vi "populate db with default.vi"(0 "SQLite Connection in":refnum<class "Connection.lvclass">, 7 "input pk list":string[](array[string]), 9 "table name":string, 11 "error in":errorcluster) -> (4 "SQLite Connection out":refnum<class "Connection.lvclass">, 15 "error out":errorcluster)   [LabVIEW 2014, in "SQLite runtime.lvclass"]
uses:
  SQLite runtime.lvclass
  <vilib>/drjdpowell/SQLite Library/SQL Connection/Connection.lvclass
  <vilib>/NI/Tag Bus/table/data table.ctl
  <vilib>/drjdpowell/SQLite Library/SQL Statement/SQL Statement.lvclass/SQL Statement.ctl
  <vilib>/drjdpowell/SQLite Library/SQL Statement/Bind Integer.vi
  <vilib>/drjdpowell/SQLite Library/SQL Statement/Bind Real.vi
  <vilib>/drjdpowell/SQLite Library/SQL Statement/Bind Text.vi
  <vilib>/drjdpowell/SQLite Library/SQL Statement/Step.vi
  <vilib>/drjdpowell/SQLite Library/SQL Statement/Error Message.vi
  <vilib>/drjdpowell/SQLite Library/SQL Statement/SQL Statement.lvclass
  <vilib>/NI/Tag Bus/table/data table.lvlib
panel:
  in  "data table":T1
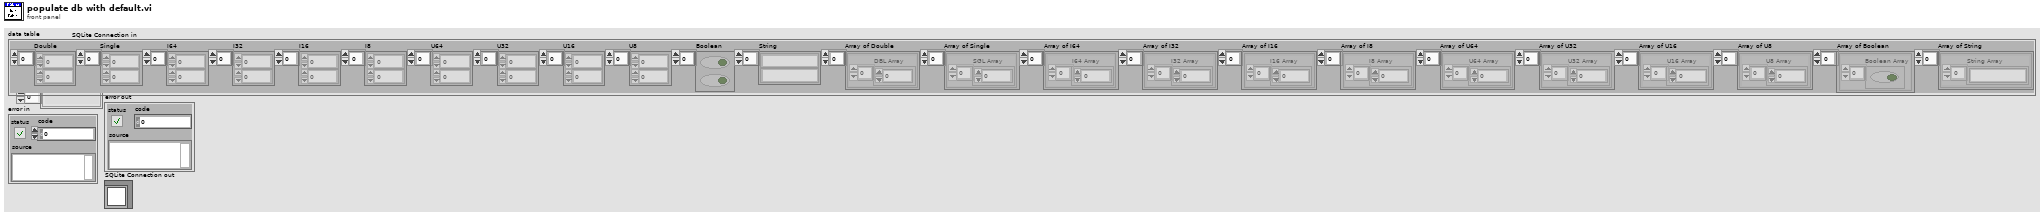
[diagram p1: front panel]
types:
  T1 = typedef "tag bus.lvlib/data table.lvlib/data table.ctl" = cluster{"Double":dbl[], "Single":sgl[], "I64":i64[], "I32":i32[], "I16":i16[], "I8":i8[], "U64":u64[], "U32":u32[], "U16":u16[], "U8":u8[], "Boolean":bool[], "String":string[], "Array of Double":cluster{"DBL Array":dbl[]}[], "Array of Single":cluster{"SGL Array":sgl[]}[], "Array of I64":cluster{"I64 Array":i64[]}[], "Array of I32":cluster{"I32 Array":i32[]}[], "Array of I16":cluster{"I16 Array":i16[]}[], "Array of I8":cluster{"I8 Array":i8[]}[], "Array of U64":cluster{"U64 Array":u64[]}[], "Array of U32":cluster{"U32 Array":u32[]}[], "Array of U16":cluster{"U16 Array":u16[]}[], "Array of U8":cluster{"U8 Array":u8[]}[], "Array of Boolean":cluster{"Boolean Array":bool[]}[], "Array of String":cluster{"String Array":string[]}[]}
  T2 = cluster{"Str":i32, "Bool":i32, "DBL":i32, "SGL":i32, "I64":i32, "I16":i32, "I32":i32, "I8":i32, "U64":i32, "U16":i32, "U32":i32, "U8":i32}
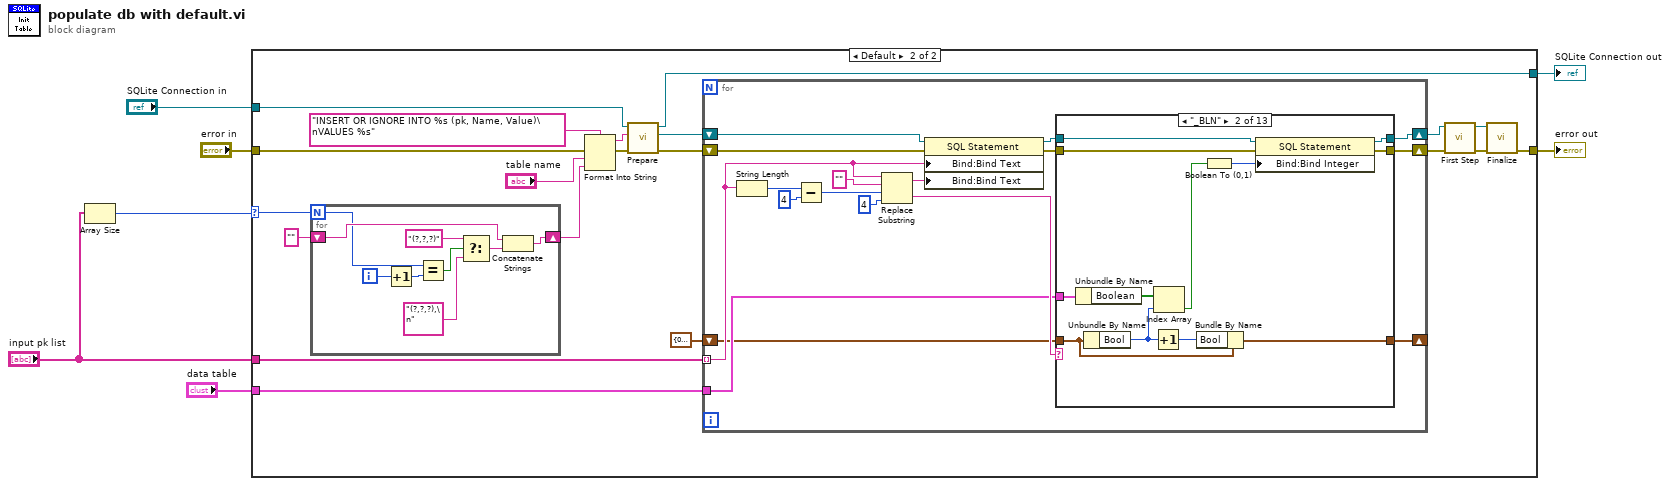
[diagram p0: block diagram]
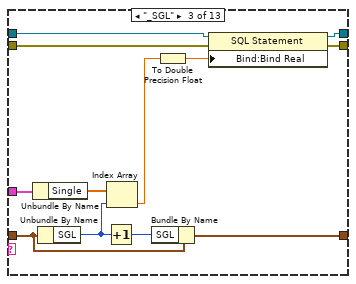
[diagram p4: hidden frame]
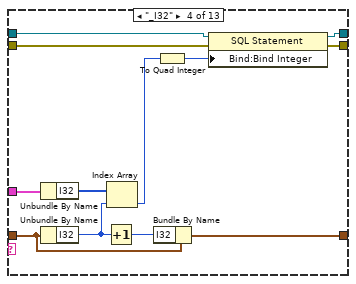
[diagram p5: hidden frame]
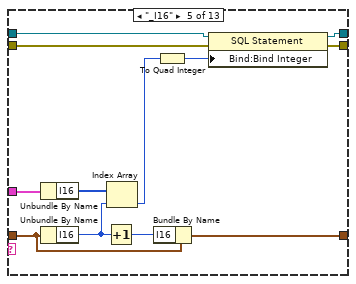
[diagram p6: hidden frame]
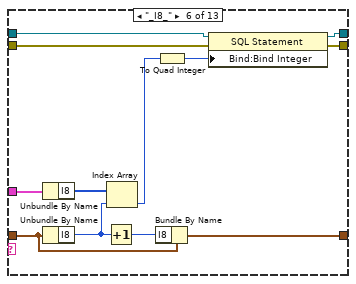
[diagram p7: hidden frame]
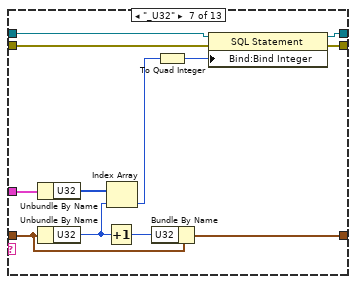
[diagram p8: hidden frame]
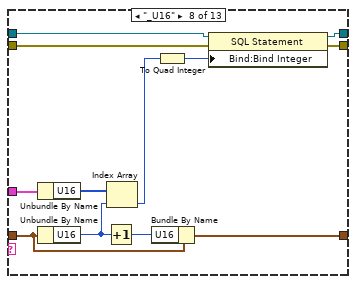
[diagram p9: hidden frame]
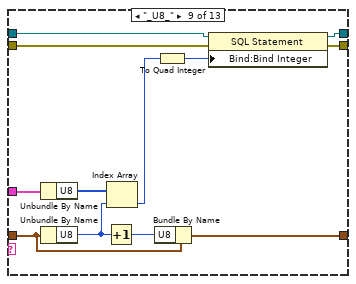
[diagram p10: hidden frame]
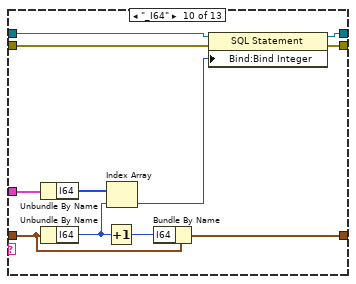
[diagram p11: hidden frame]
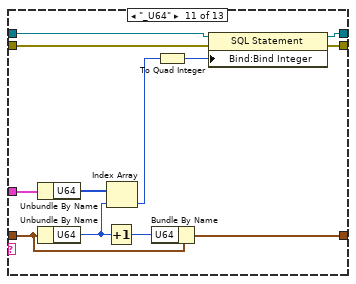
[diagram p12: hidden frame]
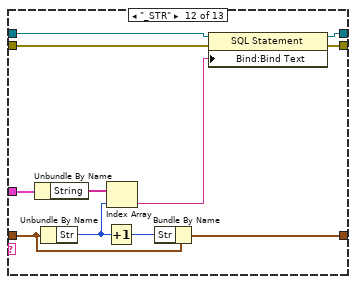
[diagram p13: hidden frame]
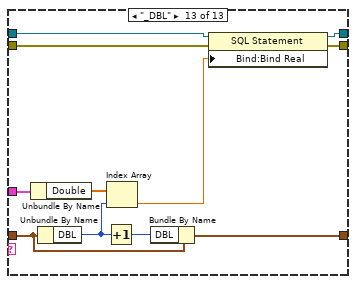
[diagram p14: hidden frame]
diagram:
  n1 = Array Size(array="input pk list") -> (size(s)=w7:i32)
  n2 = case shown="Default" w7 {
    selector: w7 -> [_ w29]
    tunnel: "SQLite Connection in" -> [w8 w25]
    tunnel: "data table" -> [_ w16]
    tunnel: "input pk list" -> [_ w19]
    tunnel: [w9 w12] -> w3
    tunnel: "error in" -> [w9 w11]
    tunnel: [w8 w10] -> w1
    frame 0 {
    }
    frame Default {
      n3 = for {
        N: w29 -> [w196]
        shift-right: [w199] -> w26
        shift-left: "" -> [w198]
        i -> [w197]
        n4 = Increment(x=w197) -> (x+1=w191:i32)
        n5 = Equal?(x=w196, y=w191) -> (x = y?=w195:bool)
        n6 = Select(t="(?,?,?)" ("string"), s=w195, f="(?,?,?),\n" ("string")) -> (s? t:f=w192:string)
        n7 = Concatenate Strings(w198, w192) -> (w199:string)
      }
      n8 = Format Into String(format string="INSERT OR IGNORE INTO %s (pk, Name, Value)\nVALUES %s" ("delimiter (Tab)"), error in=w11, "table name", w26) -> (resulting string=w23:string, error out=w17:errorcluster)  [unwired: 1 in]
      n9 = call <vilib>:"Prepare.vi"("error in (no error)"=w17, "SQL"=w23, "SQLite Connection in"=w25) -> ("error out"=w18:errorcluster, "SQL Statement out"=w20:refnum<class "SQL Statement.lvclass">, "SQLite Connection out"=w10:refnum<class "Connection.lvclass">)  [unwired: 4 in, 2 out]
      n10 = for {
        shift-right: [w42] -> w22
        shift-left: w20 -> [w46]
        tunnel: w19 -> [w35] mode=indexing
        shift-right: [w41] -> w14
        shift-left: w18 -> [w45]
        tunnel: w16 -> [w32]
        shift-right: [w30] -> _
        shift-left: T2 {"Str"=0, "Bool"=0, "DBL"=0, "SGL"=0, "I64"=0, "I16"=0, "I32"=0, "I8"=0, "U64"=0, "U16"=0, "U32"=0, "U8"=0} -> [w31]
        n11 = String Length(string=w35) -> (length=w40:i32)
        n12 = Subtract(x=w40, y=4) -> (x-y=w38:i32)
        n13 = Replace Substring(2:4 ("length (len. of substring)"), 3:w38, 4:"" ("substring (\"\")"), 5:w35) -> (0:w34:string, 1:w33:string)
        n14 = property class="SQL Statement"(reference=w46, error in=w45, "Bind:Bind Text"=w35, "Bind:Bind Text"=w33) -> (reference out=w44:refnum<class "SQL Statement.lvclass">, error out=w43:errorcluster)
        n15 = case shown="\"_BLN\"" w34 {
          tunnel: w44 -> [w48 w61 w73 w85 w97 w109 w121 w133 w145 w156 w168 w179 w190]
          tunnel: w43 -> [w49 w60 w72 w84 w96 w108 w120 w132 w144 w155 w167 w178 w189]
          tunnel: [w48 w59 w71 w83 w95 w107 w119 w131 w143 w154 w166 w177 w188] -> w42
          tunnel: [w49 w58 w70 w82 w94 w106 w118 w130 w142 w153 w165 w176 w187] -> w41
          tunnel: w32 -> [_ w57 w69 w81 w93 w105 w117 w129 w141 w152 w164 w175 w186]
          tunnel: w31 -> [w47 w54 w66 w78 w90 w102 w114 w126 w138 w149 w161 w171 w183]
          tunnel: [w47 w52 w64 w76 w88 w100 w112 w124 w136 w147 w159 w169 w181] -> w30
          frame Default {
          }
          frame "_BLN" {
            n16 = Unbundle By Name(w57) -> ("Boolean"=w56:bool[])
            n17 = Unbundle By Name(w54) -> ("Bool"=w55:i32)
            n18 = Increment(x=w55) -> (x+1=w53:i32)
            n19 = Index Array(array=w56, index=w55) -> (element=w51:bool)
            n20 = Bundle By Name(cluster=w54, "Bool"=w53) -> (w52:T2)
            n21 = Boolean To (0,1)(Boolean=w51) -> (0, 1=w50:i16)
            n22 = property class="SQL Statement"(reference=w61, error in=w60, "Bind:Bind Integer"=w50) -> (reference out=w59:refnum<class "SQL Statement.lvclass">, error out=w58:errorcluster)
          }
          frame "_SGL" {
            n23 = Unbundle By Name(w69) -> ("Single"=w68:sgl[])
            n24 = Unbundle By Name(w66) -> ("SGL"=w67:i32)
            n25 = Increment(x=w67) -> (x+1=w65:i32)
            n26 = Index Array(array=w68, index=w67) -> (element=w63:sgl)
            n27 = Bundle By Name(cluster=w66, "SGL"=w65) -> (w64:T2)
            n28 = To Double Precision Float(number=w63) -> (double precision float=w62:dbl)
            n29 = property class="SQL Statement"(reference=w73, error in=w72, "Bind:Bind Real"=w62) -> (reference out=w71:refnum<class "SQL Statement.lvclass">, error out=w70:errorcluster)
          }
          frame "_I32" {
            n30 = Unbundle By Name(w81) -> ("I32"=w80:i32[])
            n31 = Unbundle By Name(w78) -> ("I32"=w79:i32)
            n32 = Increment(x=w79) -> (x+1=w77:i32)
            n33 = Index Array(array=w80, index=w79) -> (element=w75:i32)
            n34 = Bundle By Name(cluster=w78, "I32"=w77) -> (w76:T2)
            n35 = To Quad Integer(1:w75) -> (0:w74:i64)
            n36 = property class="SQL Statement"(reference=w85, error in=w84, "Bind:Bind Integer"=w74) -> (reference out=w83:refnum<class "SQL Statement.lvclass">, error out=w82:errorcluster)
          }
          frame "_I16" {
            n37 = Unbundle By Name(w93) -> ("I16"=w92:i16[])
            n38 = Unbundle By Name(w90) -> ("I16"=w91:i32)
            n39 = Increment(x=w91) -> (x+1=w89:i32)
            n40 = Index Array(array=w92, index=w91) -> (element=w87:i16)
            n41 = Bundle By Name(cluster=w90, "I16"=w89) -> (w88:T2)
            n42 = To Quad Integer(1:w87) -> (0:w86:i64)
            n43 = property class="SQL Statement"(reference=w97, error in=w96, "Bind:Bind Integer"=w86) -> (reference out=w95:refnum<class "SQL Statement.lvclass">, error out=w94:errorcluster)
          }
          frame "_I8_" {
            n44 = Unbundle By Name(w105) -> ("I8"=w104:i8[])
            n45 = Unbundle By Name(w102) -> ("I8"=w103:i32)
            n46 = Increment(x=w103) -> (x+1=w101:i32)
            n47 = Index Array(array=w104, index=w103) -> (element=w99:i8)
            n48 = Bundle By Name(cluster=w102, "I8"=w101) -> (w100:T2)
            n49 = To Quad Integer(1:w99) -> (0:w98:i64)
            n50 = property class="SQL Statement"(reference=w109, error in=w108, "Bind:Bind Integer"=w98) -> (reference out=w107:refnum<class "SQL Statement.lvclass">, error out=w106:errorcluster)
          }
          frame "_U32" {
            n51 = Unbundle By Name(w117) -> ("U32"=w116:u32[])
            n52 = Unbundle By Name(w114) -> ("U32"=w115:i32)
            n53 = Increment(x=w115) -> (x+1=w113:i32)
            n54 = Index Array(array=w116, index=w115) -> (element=w111:u32)
            n55 = Bundle By Name(cluster=w114, "U32"=w113) -> (w112:T2)
            n56 = To Quad Integer(1:w111) -> (0:w110:i64)
            n57 = property class="SQL Statement"(reference=w121, error in=w120, "Bind:Bind Integer"=w110) -> (reference out=w119:refnum<class "SQL Statement.lvclass">, error out=w118:errorcluster)
          }
          frame "_U16" {
            n58 = Unbundle By Name(w129) -> ("U16"=w128:u16[])
            n59 = Unbundle By Name(w126) -> ("U16"=w127:i32)
            n60 = Increment(x=w127) -> (x+1=w125:i32)
            n61 = Index Array(array=w128, index=w127) -> (element=w123:u16)
            n62 = Bundle By Name(cluster=w126, "U16"=w125) -> (w124:T2)
            n63 = To Quad Integer(1:w123) -> (0:w122:i64)
            n64 = property class="SQL Statement"(reference=w133, error in=w132, "Bind:Bind Integer"=w122) -> (reference out=w131:refnum<class "SQL Statement.lvclass">, error out=w130:errorcluster)
          }
          frame "_U8_" {
            n65 = Unbundle By Name(w141) -> ("U8"=w140:u8[])
            n66 = Unbundle By Name(w138) -> ("U8"=w139:i32)
            n67 = Increment(x=w139) -> (x+1=w137:i32)
            n68 = Index Array(array=w140, index=w139) -> (element=w135:u8)
            n69 = Bundle By Name(cluster=w138, "U8"=w137) -> (w136:T2)
            n70 = To Quad Integer(1:w135) -> (0:w134:i64)
            n71 = property class="SQL Statement"(reference=w145, error in=w144, "Bind:Bind Integer"=w134) -> (reference out=w143:refnum<class "SQL Statement.lvclass">, error out=w142:errorcluster)
          }
          frame "_I64" {
            n72 = Unbundle By Name(w152) -> ("I64"=w151:i64[])
            n73 = Unbundle By Name(w149) -> ("I64"=w150:i32)
            n74 = Increment(x=w150) -> (x+1=w148:i32)
            n75 = Index Array(array=w151, index=w150) -> (element=w146:i64)
            n76 = Bundle By Name(cluster=w149, "I64"=w148) -> (w147:T2)
            n77 = property class="SQL Statement"(reference=w156, error in=w155, "Bind:Bind Integer"=w146) -> (reference out=w154:refnum<class "SQL Statement.lvclass">, error out=w153:errorcluster)
          }
          frame "_U64" {
            n78 = Unbundle By Name(w164) -> ("U64"=w163:u64[])
            n79 = Unbundle By Name(w161) -> ("U64"=w162:i32)
            n80 = Increment(x=w162) -> (x+1=w160:i32)
            n81 = Index Array(array=w163, index=w162) -> (element=w158:u64)
            n82 = Bundle By Name(cluster=w161, "U64"=w160) -> (w159:T2)
            n83 = To Quad Integer(1:w158) -> (0:w157:i64)
            n84 = property class="SQL Statement"(reference=w168, error in=w167, "Bind:Bind Integer"=w157) -> (reference out=w166:refnum<class "SQL Statement.lvclass">, error out=w165:errorcluster)
          }
          frame "_STR" {
            n85 = Unbundle By Name(w175) -> ("String"=w174:string[])
            n86 = Unbundle By Name(w171) -> ("Str"=w172:i32)
            n87 = Increment(x=w172) -> (x+1=w170:i32)
            n88 = Index Array(array=w174, index=w172) -> (element=w173:string)
            n89 = Bundle By Name(cluster=w171, "Str"=w170) -> (w169:T2)
            n90 = property class="SQL Statement"(reference=w179, error in=w178, "Bind:Bind Text"=w173) -> (reference out=w177:refnum<class "SQL Statement.lvclass">, error out=w176:errorcluster)
          }
          frame "_DBL" {
            n91 = Unbundle By Name(w186) -> ("Double"=w185:dbl[])
            n92 = Unbundle By Name(w183) -> ("DBL"=w184:i32)
            n93 = Increment(x=w184) -> (x+1=w182:i32)
            n94 = Index Array(array=w185, index=w184) -> (element=w180:dbl)
            n95 = Bundle By Name(cluster=w183, "DBL"=w182) -> (w181:T2)
            n96 = property class="SQL Statement"(reference=w190, error in=w189, "Bind:Bind Real"=w180) -> (reference out=w188:refnum<class "SQL Statement.lvclass">, error out=w187:errorcluster)
          }
        }
      }
      n97 = call <vilib>:"First Step.vi"("error in (no error)"=w14, "SQL Statement in"=w22) -> ("error out"=w13:errorcluster, "SQL Statement out"=w21:refnum<class "SQL Statement.lvclass">)  [unwired: 7 in, 1 out]
      n98 = call <vilib>:"Finalize.vi"("error in (no error)"=w13, "SQL Statement in"=w21) -> ("error out"=w12:errorcluster)  [unwired: 9 in]
    }
  }
  "error out" <- w3
  "SQLite Connection out" <- w1
